vi "Set Initialization Data - DataSave.vi"(8 "error in":errorcluster, 11 "DataAcquire Worker in":refnum<class "DataAcquire Worker.lvclass">) -> (0 "error out":errorcluster, 3 "DataAcquire Worker out":refnum<class "DataAcquire Worker.lvclass">)   [LabVIEW 2018, in "DataAcquire Worker.lvclass"]
doc: "Sets the initialization data of a statically linked subWorker."
uses:
  DataAcquire Worker.lvclass
  DataSave Worker/Initialization Data.ctl
  DataAcquire Worker.lvclass/DataAcquire Worker.ctl
  DataSave Worker/DataSave Worker.lvclass
  D:/Program Files (x86)/National Instruments/LabVIEW 2018/vi.lib/addons/_Workers/Library/Classes/Worker/Worker.lvclass
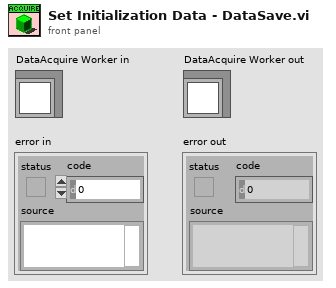
[diagram p1: front panel]
types:
  T1 = typedef "DataSave Worker.lvclass/Initialization Data.ctl" = cluster{"String":string}
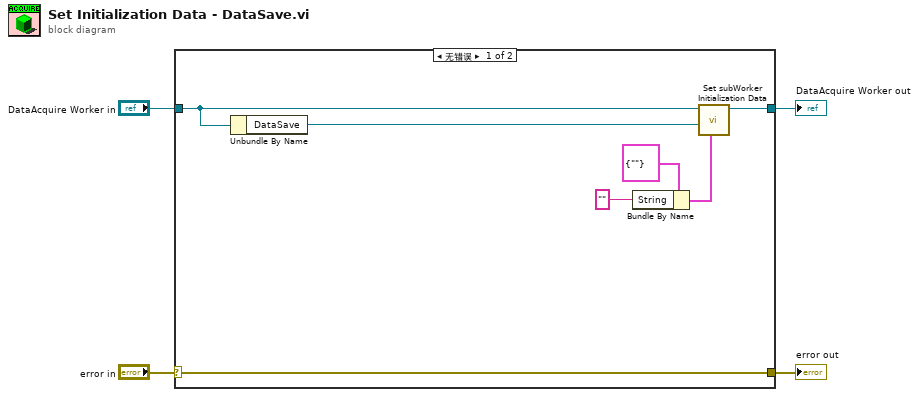
[diagram p0: block diagram]
diagram:
  n1 = case shown="无错误" "error in" {
    selector: "error in" -> [w11 w13]
    tunnel: [w11 w13] -> w3
    tunnel: [w9 w12] -> w2
    tunnel: "DataAcquire Worker in" -> [w8 w12]
    frame No Error {
      n2 = Unbundle By Name(w8) -> ("DataSave"=w10:refnum<class "DataSave Worker.lvclass">)
      n3 = Bundle By Name(cluster=T1 {"String"=""} ("Initialization Data"), "String"="" ("Placeholder")) -> (w6:T1)
      n4 = call-dynamic "Set subWorker Initialization Data.vi"("Initialization Data"=w6, "subWorker"=w10, "Worker"=w8) -> ("Worker out"=w9:refnum<class "DataAcquire Worker.lvclass">)  [unwired: 8 in]
    }
    frame Error {
    }
  }
  "error out" <- w3
  "DataAcquire Worker out" <- w2
